vi "ConfigSysClk.vi"(8 "error in (no error)":errorcluster, 11 "PXI_MultiTrig in":refnum<class "PXI_MultiTrig.lvclass">) -> (0 "error out":errorcluster, 3 "PXI_MultiTrig out":refnum<class "PXI_MultiTrig.lvclass">)   [LabVIEW 2018, in "SyncPlugins.lvlib" / "PXI_MultiTrig.lvclass"]
uses:
  PXI_MultiTrig.lvclass
  PXI_MultiTrig.lvclass/PXI_MultiTrig.ctl
  Accessors/Write SysHandle.vi
  Accessors/Write SysRef.vi
  Accessors/Read SyncWindowsClock.vi
  <vilib>/Utility/error.llb/Error Cluster From Error Code.vi
  <vilib>/ErrorRing/Error Ring.xnode
  <vilib>/nisyscfg/nisyscfg.lvlib
  <resource>/objmgr/niMIDebugSession.rc
  <resource>/objmgr/nisysapi.rc
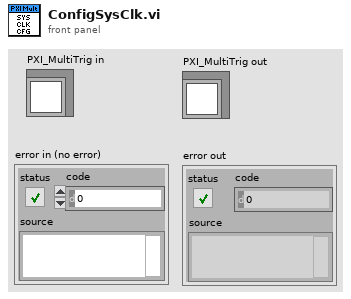
[diagram p1: front panel]
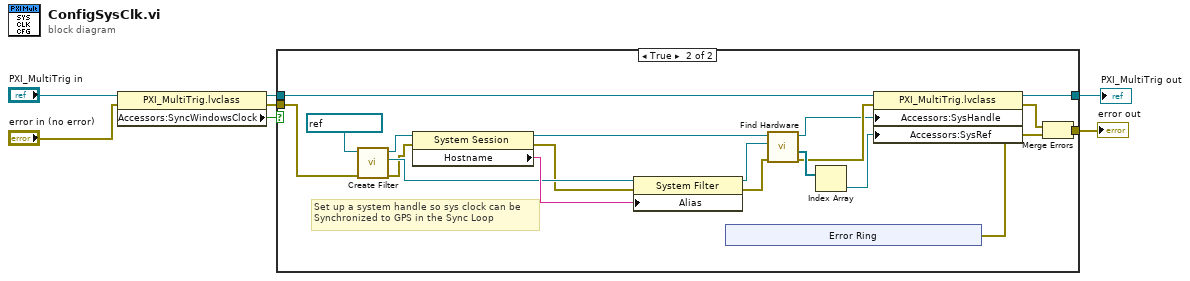
[diagram p0: block diagram]
diagram:
  n1 = property class="PXI_MultiTrig.lvclass"(reference="PXI_MultiTrig in", error in="error in (no error)") -> (reference out=w5:refnum<class "PXI_MultiTrig.lvclass">, error out=w2:errorcluster, "Accessors:SyncWindowsClock"=w1:bool)
  n2 = case shown="True" w1 {
    tunnel: [w8 w18] -> w7
    tunnel: w5 -> [w8 w15]
    tunnel: [w9 w14] -> w3
    tunnel: w2 -> [w9 w12]
    frame False {
    }
    frame True {
      # "Set up a system handle so sys clock can be\nSynchronized to GPS in the Sync Loop"
      n3 = call <vilib>:"Create Filter.vi"("error in (no error)"=w12, "Session in"=refnum<k21> "localhost") -> ("error out"=w20:errorcluster, "Filter out"=w21:refnum<k20>, "Session out"=w23:refnum<k21>)  [unwired: 7 in]
      n4 = property class="System Session"(reference=w23, error in=w20) -> (reference out=w25:refnum<k21>, error out=w19:errorcluster, "Hostname"=w24:string)
      n5 = property class="System Filter"(reference=w21, error in=w19, "Alias"=w24) -> (reference out=w26:refnum<k20>, error out=w27:errorcluster)
      n6 = xnode "Error Ring"() -> ("error out"=w13:errorcluster)
      n7 = call <vilib>:"Find Hardware.vi"("error in (no error)"=w27, "Filter in"=w26, "Session in"=w25) -> ("error out"=w17:errorcluster, "Resources out"=w28:refnum<k20>[], "Session out"=w10:refnum<k21>)  [unwired: 5 in, 1 out]
      n8 = Index Array(array=w28) -> (element=w11:refnum<k20>)  [unwired: 1 in]
      n9 = property class="PXI_MultiTrig.lvclass"(reference=w15, error in=w17, "Accessors:SysHandle"=w10, "Accessors:SysRef"=w11) -> (reference out=w18:refnum<class "PXI_MultiTrig.lvclass">, error out=w16:errorcluster)
      n10 = Merge Errors(w16, w13) -> (w14:errorcluster)
    }
  }
  "error out" <- w3
  "PXI_MultiTrig out" <- w7
